vi "Tool Q LEIN High G Stopp.vi"(0 "Controller ID":u8=42, 11 "error in (no error)":errorcluster) -> (4 "LEIN custom reply Q":T1, 15 "error out":errorcluster)   [LabVIEW 2011]
uses:
  LEINmaster/Defenitions/LEIN custom reply Q.ctl
  LEINmaster/Defenitions/LEIN Reply Holder.ctl
  LEINmaster/Defenitions/LEIN CMD Cluster.ctl
  LEINmaster/Defenitions/LEIN CMD List.ctl
  LEINmaster/Defenitions/LEIN Structure variations.ctl
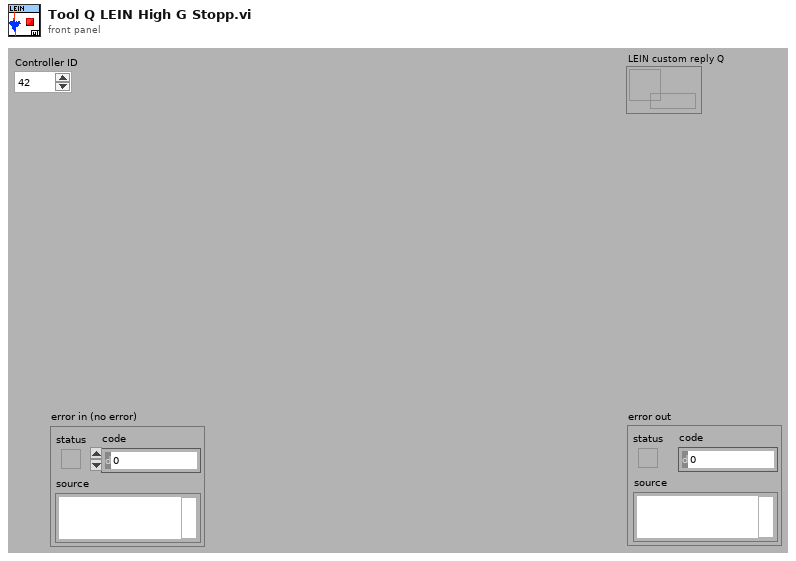
[diagram p1: front panel]
types:
  T1 = typedef "LEIN custom reply Q.ctl" = refnum<queue>
  T2 = typedef "LEIN Structure variations.ctl" = enum16{"LEIN08", "LEIN31", "LEIN63"}
  T3 = typedef "LEIN CMD Cluster.ctl" = cluster{"SID":u8, "ANF":bool, "CMD":T4, "DATA":u8[]}
  T4 = typedef "LEIN CMD List.ctl" = enum8{"ACTI", "TASK", "RES0", "STAT", "RES1", "RES2", "RES3", "USER"}
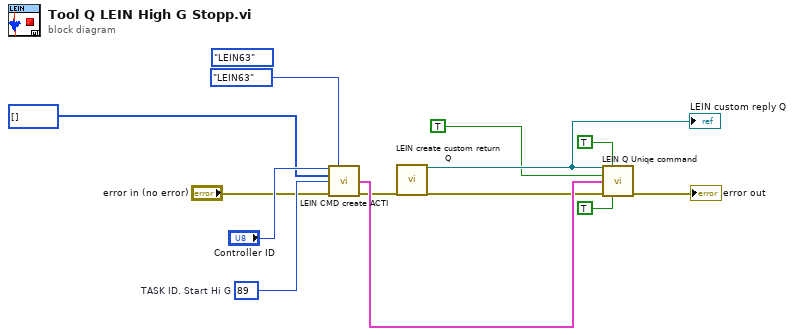
[diagram p0: block diagram]
diagram:
  (unwired) LEIN_Structure_variations."LEIN63" ("LEIN Variation")
  w11 = u8 89  # TASK ID. Start Hi G
  n1 = call "LEIN CMD create ACTI.vi"("SID"="Controller ID", "LEIN Variation"=LEIN_Structure_variations."LEIN63", "Data"=u8[] [], "ACTI ID"=w11, "error in (no error)"="error in (no error)") -> ("CMD"=w6:T3, "error out"=w5:errorcluster)  [unwired: 9 in]
  n2 = call "LEIN create custom return Q.vi"("error in (no error)"=w5) -> ("LEIN custom reply Q"=w4:T1, "error out"=w3:errorcluster)  [unwired: 13 in]
  "LEIN custom reply Q" <- w4
  n3 = call "LEIN Q Uniqe command.vi"("LEIN custom reply Q"=w4, "Retry on err (F)"=TRUE, "Custom Q(F)"=TRUE, "CMD"=w6, "error in"=w3, "priority(F)"=TRUE) -> ("error out"=→"error out":errorcluster)  [unwired: 9 in]
